vi "dosing control.vi"() -> ()   [LabVIEW 2012]
uses:
  Instance           1 22Saved   dosing control .vi
  Instance           2 22Saved   dosing control .vi
panel:
  in  "?":bool
  out "Overdosing":bool
  in  "Dosing Limit":dbl=20.0 format="%.2f"
  in  "Base Pressure":dbl=6.47 format="%.2f"
  out "Waveform Chart":dynamicdata(graph)=[{"t0"=timestamp(3248038146.94875 s since 1904-01-01), "dt"=0.1, "Y"=[7.375785452699056], "attributes"=variant("NI_ChannelName"=variant(string "Voltage (Mean)"), "NI_OriginalChannelName"=variant(string "Voltage"), "NI_UnitDescription"=variant(string "Volts"))}]
  out "Pressure":dbl format="%.2f"
  out "Oxygen (L)":dbl format="%.1f"
  out "High Pressure":bool
  in  "Upper Pressure Limit":dbl=10.0 format="%.2f"
  in  "?":bool
  # "Dosed Amount"
  # "start"
  # "stop"
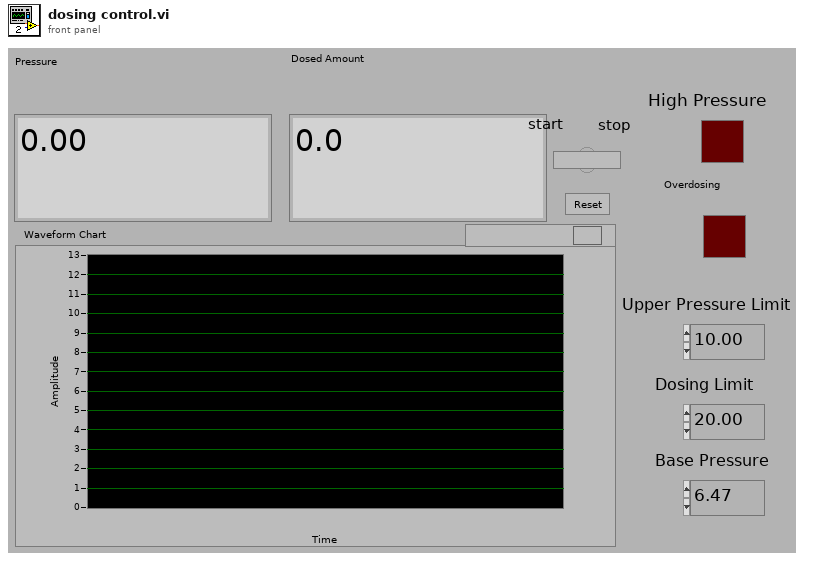
[diagram p1: front panel]
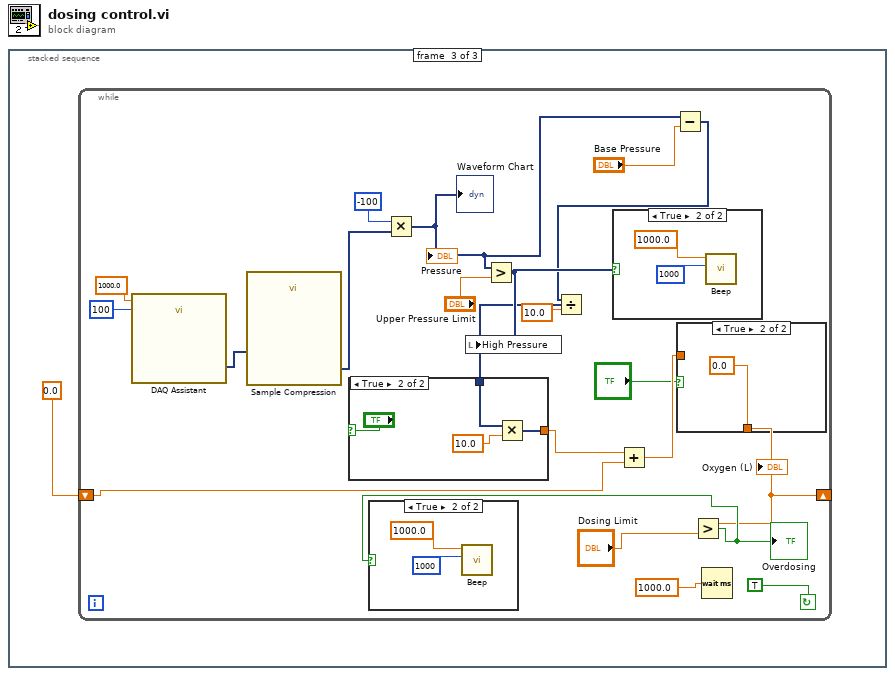
[diagram p0: block diagram]
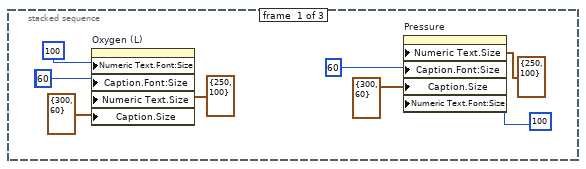
[diagram p2: hidden frame]
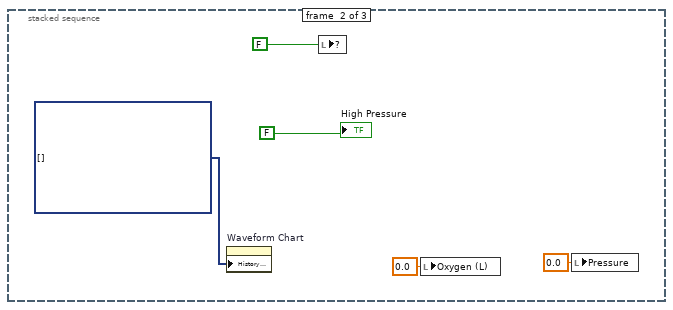
[diagram p3: hidden frame]
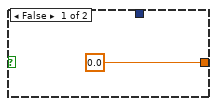
[diagram p6: hidden frame]
diagram:
  n1 = stacked-sequence {
    frame #0 {
      (unwired) u32 60 ("Numeric Text.Font:Size")
      n2 = property on="Oxygen (L)" class="DigNum (strict)"("Numeric Text.Font:Size"=u32 100, "Caption.Font:Size"=u32 60 ("Numeric Text.Font:Size"), "Numeric Text.Size"=cluster{"Width":u32, "Height":u32} {"Width"=250, "Height"=100}, "Caption.Size"=cluster{"Width":u32, "Height":u32} {"Width"=300, "Height"=60} ("Label.Size")) -> ()  [unwired: 2 in, 2 out]
      n3 = property on="Pressure" class="DigNum (strict)"("Numeric Text.Size"=cluster{"Width":u32, "Height":u32} {"Width"=250, "Height"=100} ("Numeric Text.Bounds"), "Caption.Font:Size"=u32 60 ("Numeric Text.Font:Size"), "Caption.Size"=cluster{"Width":u32, "Height":u32} {"Width"=300, "Height"=60} ("Label.Size"), "Numeric Text.Font:Size"=100) -> ()  [unwired: 2 in, 2 out]
    }
    frame #1 {
      n4 = property on="Waveform Chart" class="WFChart (strict)"("History Data"=dynamicdata[] []) -> ()  [unwired: 2 in, 2 out]
      n5 = local write item#?(FALSE ("Operation Switch")) -> ()
      n6 = local write "Oxygen (L)"(0.0 ("Oxygen (L)")) -> ()
      n7 = local write "Pressure"(0.0 ("Pressure")) -> ()
      "High Pressure" <- FALSE
    }
    frame #2 {
      n8 = while {
        shift-left: 0.0 -> [w18]
        shift-right: [w16] -> _
        stop <- TRUE continue-if-true
        n9 = call "DAQ Assistant"("rate"=1000.0, "number of samples"=100) -> ("data"=w29:dynamicdata)  [unwired: 15 in, 2 out]
        n10 = call "Sample Compression"("Signals"=w29) -> ("Mean"=w28:dynamicdata)  [unwired: 8 in, 2 out]
        n11 = Multiply(x=-100, y=w28) -> (x*y=w24:dynamicdata)
        "Pressure" <- w24
        "Waveform Chart" <- w24
        n12 = Greater?(x=w24, y="Upper Pressure Limit") -> (0:w35:dynamicdata)
        n13 = local write "High Pressure"(w35) -> ()
        n14 = case shown="True" w35 {
          frame False {
          }
          frame True {
            n15 = call <vilib>:"Beep.vi"("duration (msec)"=i16 1000 ("duration (msec) - ignored"), "frequency (Hz)"=1000.0 ("frequency (Hz) - ignored")) -> ()  [unwired: 10 in]
          }
        }
        n16 = Subtract(x=w24, y="Base Pressure") -> (x-y=w22:dynamicdata)
        n17 = Divide(x=w22, y=10.0) -> (x/y=w31:dynamicdata)
        n18 = case shown="True" "?" {
          tunnel: [0.0 w42] -> w19
          tunnel: w31 -> [_ w44]
          frame False {
            (unwired) 0.0
          }
          frame True {
            n19 = Multiply(x=w44, y=10.0) -> (x*y=w42:dynamicdata)
          }
        }
        n20 = Add(x=w19, y=w18) -> (x+y=w17:dbl)
        n21 = case shown="True" "?" {
          tunnel: w17 -> [w37 _]
          tunnel: [w37 0.0 ("y")] -> w16
          frame False {
          }
          frame True {
          }
        }
        "Oxygen (L)" <- w16
        n22 = Greater?(x=w16, y="Dosing Limit") -> (0:w20:bool)
        "Overdosing" <- w20
        n23 = case shown="True" w20 {
          frame False {
          }
          frame True {
            n24 = call <vilib>:"Beep.vi"("duration (msec)"=i16 1000 ("duration (msec) - ignored"), "frequency (Hz)"=1000.0 ("frequency (Hz) - ignored")) -> ()  [unwired: 10 in]
          }
        }
        n25 = Wait (ms)(milliseconds to wait=1000.0 ("y")) -> ()  [unwired: 1 out]
      }
    }
  }
